vi "output_fgv.vi"(2 "single state":bool=TRUE, 3 "index":i32, 4 "error in":errorcluster, 5 "Line(s)":tag="Dev8/port0/line0:7", 6 "action":T1=enum."set values", 7 "simulate":bool=TRUE) -> (0 "error out":errorcluster, 1 "current valve states":bool[](array[boolean]))   [LabVIEW 2016]
uses:
  output.ctl
panel:
  out "simulate check":bool
  in  "states":bool[](array[boolean])=[FALSE, FALSE, FALSE, FALSE, FALSE, FALSE, FALSE, FALSE]
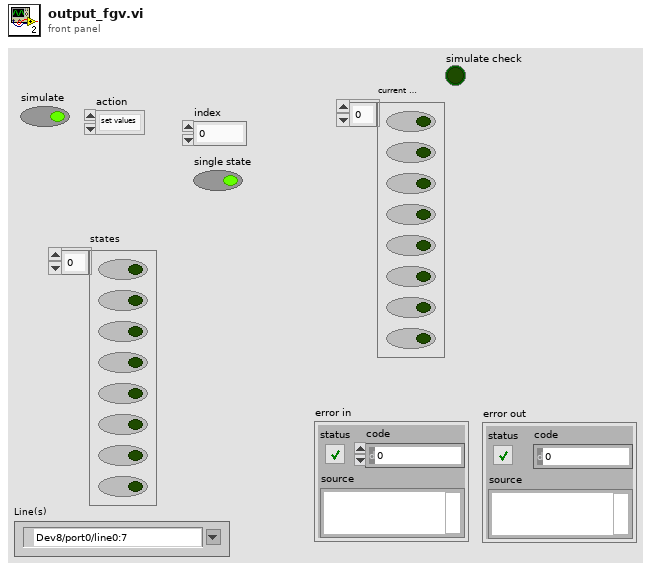
[diagram p1: front panel]
types:
  T1 = typedef "output.ctl" = enum16{"init", "set values", "apply", "read"}
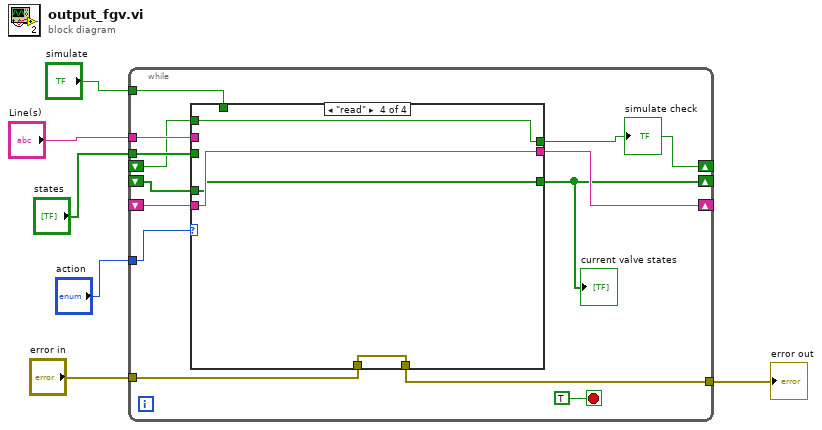
[diagram p0: block diagram]
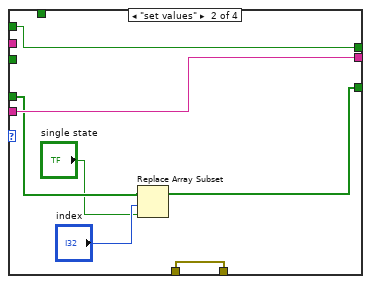
[diagram p3: hidden frame]
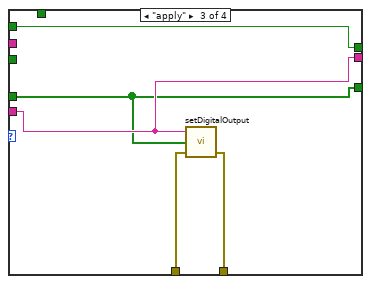
[diagram p4: hidden frame]
diagram:
  n1 = while {
    shift-right: [w9] -> _
    shift-left: _ -> [w16]
    tunnel: "Line(s)" -> [w15]
    tunnel: "simulate" -> [w11]
    tunnel: "action" -> [w18]
    shift-right: [w14] -> _
    shift-left: _ -> [w13]
    tunnel: "states" -> [w17]
    shift-right: [w10] -> _
    shift-left: _ -> [w12]
    tunnel: "error in" -> [w8]
    tunnel: [w7] -> w1
    stop <- TRUE stop-if-true
    n2 = case shown="\"read\"" w18 {
      tunnel: w17 -> [w23 _ _ _]
      tunnel: [w23 w25 w33 w38] -> w9
      tunnel: w16 -> [_ w28 w33 w38]
      tunnel: w15 -> [w22 _ _ _]
      tunnel: [w22 w29 w34 w39] -> w14
      tunnel: w13 -> [_ w29 w34 w39]
      tunnel: w12 -> [_ w30 w35 w37]
      tunnel: w11 -> [w21 _ _ _]
      tunnel: [w21 w30 w35 w37] -> w10
      tunnel: w8 -> [w20 w24 w32 w36]
      tunnel: [w20 w24 w31 w36] -> w7
      frame "init", Default {
      }
      frame "set values" {
        n3 = Replace Array Subset(array=w28, new element="single state", index="index") -> (w25:bool[])
      }
      frame "apply" {
        n4 = call "setDigitalOutput.vi"("error in"=w32, "data"=w33, "Line(s)"=w34) -> ("error out"=w31:errorcluster)  [unwired: 2 in]
      }
      frame "read" {
      }
    }
    "current valve states" <- w9
    "simulate check" <- w10
  }
  "error out" <- w1
